vi "shippingM100.vi"() -> ()   [LabVIEW 2012]
uses:
  <vilib>/addons/database/Auxilliary.llb/DB Tools Cursor Type.ctl
  <vilib>/Utility/NIReport.llb/NI_report.lvclass
  <vilib>/addons/database/Connection.llb/DB Tools Open Connec (Path).vi
  <vilib>/addons/database/Connection.llb/Conn Execute.vi
  <vilib>/addons/database/Recordset.llb/Rec Destroy - Connection.vi
  <vilib>/addons/database/NI_Database_API.lvlib
panel:
  out "error out 2":errorcluster
  out "error out 4":errorcluster
  out "String 3":string
  out "String 2":string
  out "appended path":path
  out "size(s)":i32
  out "error out":errorcluster
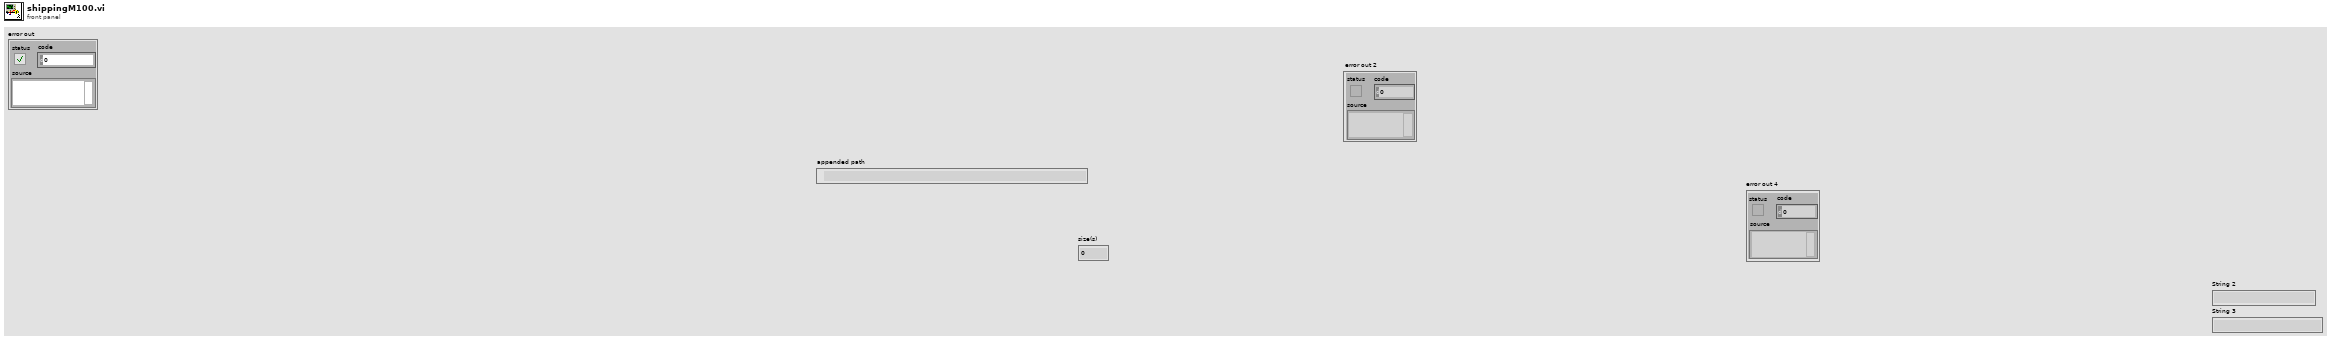
[diagram p1: front panel]
types:
  T1 = typedef "NI_Database_API.lvlib/DB Tools Cursor Type.ctl" = enum16{"forward-only", "keyset", "dynamic", "static"}
  T2 = typedef "NI_Database_API.lvlib/Conn ObjectReference.ctl" = refnum<k1>
  T3 = typedef "NI_Database_API.lvlib/Rec ObjectReference.ctl" = refnum<k1>
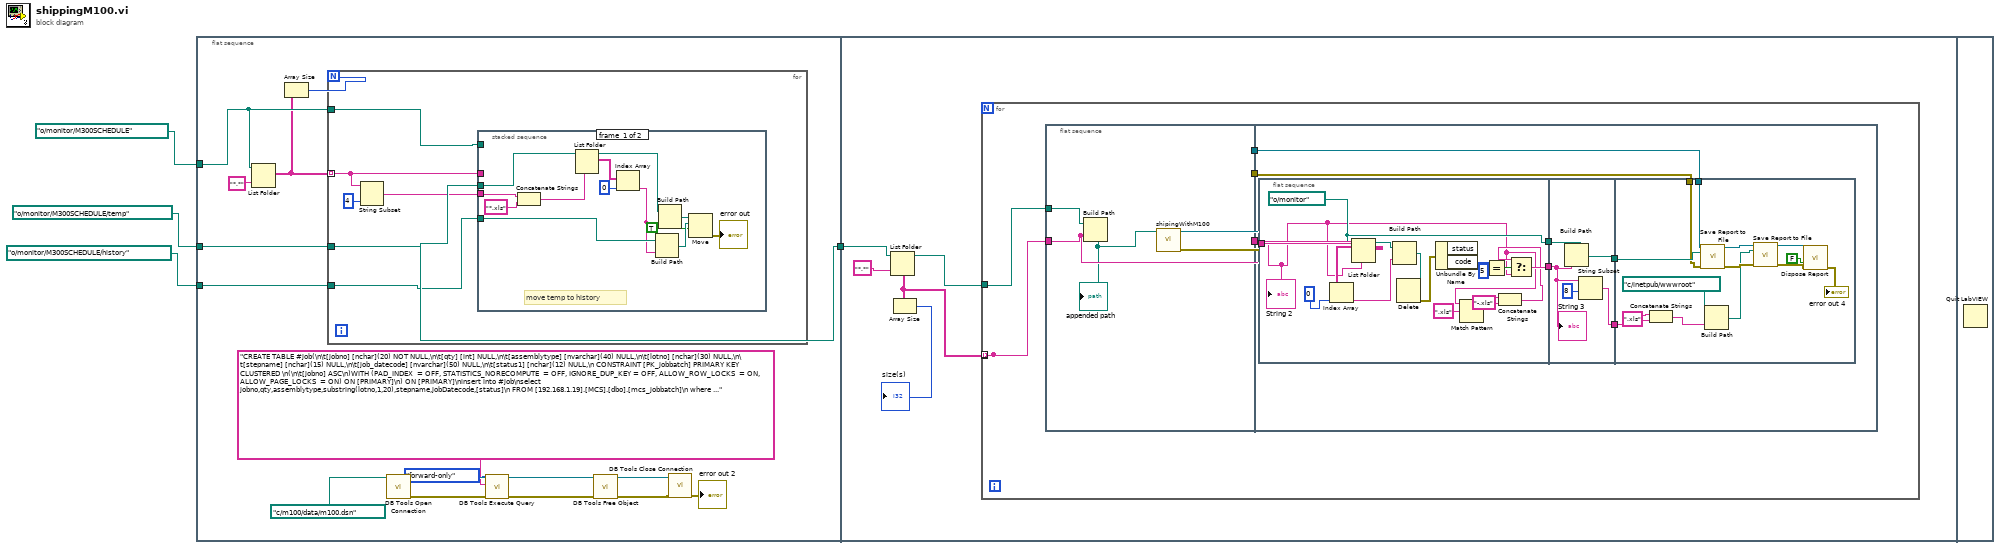
[diagram p0: block diagram]
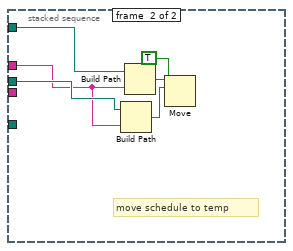
[diagram p2: hidden frame]
diagram:
  n1 = flat-sequence {
    tunnel: path "o:/monitor/M300SCHEDULE/temp" ("path") -> [w17]
    tunnel: [w17] -> w4
    tunnel: path "o:/monitor/M300SCHEDULE" ("path") -> [w19]
    tunnel: path "o:/monitor/M300SCHEDULE/history" ("path") -> [w18]
    tunnel: w4 -> [w49]
    frame #0 {
      n2 = List Folder(path=w19, pattern="*.*") -> (filenames=w15:string[])  [unwired: 2 in, 3 out]
      n3 = Array Size(array=w15) -> (size(s)=w16:i32)
      n4 = for {
        N: w16 -> [_]
        tunnel: w19 -> [w26]
        tunnel: w18 -> [w25]
        tunnel: w17 -> [w24]
        tunnel: w15 -> [w21] mode=indexing
        n5 = String Subset(string=w21, length (rest)=4 ("length (rest)")) -> (substring=w22:string)  [unwired: 1 in]
        n6 = stacked-sequence {
          tunnel: w24 -> [w35 w42]
          tunnel: w25 -> [w38 _]
          tunnel: w26 -> [_ w43]
          tunnel: w22 -> [w30 _]
          tunnel: w21 -> [_ w40]
          frame #0 {
            # "move temp to history"
            n7 = Concatenate Strings(w30, "*.xls" ("pattern")) -> (w28:string)
            n8 = List Folder(path=w35, pattern=w28) -> (path out=w34:path, filenames=w33:string[])  [unwired: 2 in, 2 out]
            n9 = Index Array(array=w33, index=0) -> (element=w31:string)
            n10 = Build Path(base path=w38, name or relative path=w31) -> (appended path=w37:path)
            n11 = Build Path(base path=w34, name or relative path=w31) -> (appended path=w39:path)
            n12 = Move(source path=w39, 9:TRUE ("overwrite (F)"), 10:w37) -> (error out=→"error out":errorcluster)  [unwired: 2 in, 2 out]
          }
          frame #1 {
            # "move schedule to temp"
            n13 = Build Path(base path=w42, name or relative path=w40) -> (appended path=w44:path)
            n14 = Build Path(base path=w43, name or relative path=w40) -> (appended path=w45:path)
            n15 = Move(source path=w45, 9:TRUE ("overwrite (F)"), 10:w44) -> ()  [unwired: 2 in, 3 out]
          }
        }
      }
      n16 = call-poly <vilib>:"DB Tools Open Connection.vi"("connection information"=path "c:/m100/data/m100.dsn") -> ("error out"=w12:errorcluster, "connection reference"=w14:T2)  [unwired: 7 in]
      n17 = call-poly <vilib>:"DB Tools Execute Query.vi"("error in (no error)"=w12, "cursor type"=DB_Tools_Cursor_Type."forward-only", "SQL query"="CREATE TABLE #job(\n\t[jobno] [nchar](20) NOT NULL,\n\t[qty] [int] NULL,\n\t[assemblytype] [nvarchar](40) NULL,\n\t[lotno] [nchar](30) NULL,\n\t[stepname] [nchar](15) NULL,\n\t[job_datecode] [nvarchar](50) NULL,\n\t[status1] [nchar](12) NULL,\n CONSTRAINT [PK_jobbatch] PRIMARY KEY CLUSTERED \n(\n\t[jobno] ASC\n)WITH (PAD_INDEX  = OFF, STATISTICS_NORECOMPUTE  = OFF, IGNORE_DUP_KEY = OFF, ALLOW_ROW_LOCKS  = ON, ALLOW_PAGE_LOCKS  = ON) ON [PRIMARY]\n) ON [PRIMARY]\ninsert into #job\nselect jobno,qty,assemblytype,substring(lotno,1,20),stepname,jobDatecode,[status]\n FROM [192.168.1.19].[MCS].[dbo].[mcs_jobbatch]\n where jobno not like '%M14110001%'\n   and lastupdatedate > 20140601", "connection reference"=w14) -> ("error out"=w11:errorcluster, "recordset reference"=w13:T3)  [unwired: 4 in]
      n18 = call-poly <vilib>:"DB Tools Free Object.vi"("error in (no error)"=w11, "recordset reference"=w13) -> ("error out"=w6:errorcluster, "connection reference"=w7:T2)  [unwired: 8 in]
      n19 = call <vilib>:"DB Tools Close Connection.vi"("error in (no error)"=w6, "connection reference"=w7) -> ("error out"=→"error out 2":errorcluster)  [unwired: 5 in]
    }
    frame #1 {
      n20 = List Folder(path=w49, pattern="*.*") -> (path out=w47:path, filenames=w46:string[])  [unwired: 2 in, 2 out]
      n21 = Array Size(array=w46) -> (size(s)=→"size(s)":i32)
      n22 = for {
        tunnel: w46 -> [w51] mode=indexing
        tunnel: [w51] -> _ mode=indexing
        tunnel: w47 -> [w55]
        n23 = flat-sequence {
          tunnel: w55 -> [w60]
          tunnel: w51 -> [w59]
          tunnel: [w59] -> w54
          tunnel: [w57] -> w53
          tunnel: [w56] -> w52
          tunnel: w54 -> [w64]
          tunnel: w53 -> [w63]
          tunnel: w52 -> [w62]
          frame #0 {
            n24 = Build Path(base path=w60, name or relative path=w59) -> (appended path=w58:path)
            "appended path" <- w58
            n25 = call "shipingWithM100.vi"("template (empty)"=w58) -> ("error out"=w56:errorcluster, "report out"=w57:refnum<class "NI_report.lvclass">)  [unwired: 9 in]
          }
          frame #1 {
            n26 = flat-sequence {
              tunnel: [w69] -> w67
              tunnel: [w71] -> w66
              tunnel: w64 -> [w68]
              tunnel: w67 -> [w88]
              tunnel: w66 -> [w87]
              tunnel: [w85] -> w65
              tunnel: [w84] -> w61
              tunnel: w65 -> [w100]
              tunnel: w63 -> [w99]
              tunnel: w62 -> [w98]
              tunnel: w61 -> [w91]
              frame #0 {
                w69 = path "o:/monitor" ("base path")
                n27 = List Folder(path=w69, pattern=w68) -> (path out=w81:path, filenames=w83:string[])  [unwired: 2 in, 2 out]
                n28 = Index Array(array=w83, index=0) -> (element=w80:string)
                n29 = Build Path(base path=w81, name or relative path=w80) -> (appended path=w79:path)
                n30 = Delete(path (use dialog)=w79) -> (error out=w78:errorcluster)  [unwired: 4 in, 2 out]
                n31 = Unbundle By Name(w78) -> ("code"=w77:i32)  [unwired: 1 out]
                n32 = Match Pattern(string=w68, regular expression=".xls") -> (match substring=w73:string)  [unwired: 1 in, 3 out]
                n33 = Equal?(x=w77, y=5) -> (x = y?=w75:bool)
                n34 = Concatenate Strings(w73, "-.xls" ("string")) -> (w70:string)
                n35 = Select(t=w70, s=w75, f=w68) -> (s? t:f=w71:string)
                "String 2" <- w68
              }
              frame #1 {
                n36 = Build Path(base path=w88, name or relative path=w87) -> (appended path=w85:path)
                n37 = String Subset(string=w87, length (rest)=8 ("length (rest)")) -> (substring=w84:string)  [unwired: 1 in]
                "String 3" <- w87
              }
              frame #2 {
                n38 = Concatenate Strings(w91, ".xls" ("string")) -> (w89:string)
                n39 = call-dynamic "Save Report to File.vi"("report in"=w99, "report file path"=w100, "error in (no error)"=w98) -> ("report out"=w95:refnum<class "NI_report.lvclass">, "error out"=w96:errorcluster)  [unwired: 11 in]
                n40 = Build Path(base path=path "c:/inetpub/wwwroot", name or relative path=w89) -> (appended path=w92:path)
                n41 = call-dynamic "Save Report to File.vi"("report in"=w95, "report file path"=w92, "error in (no error)"=w96) -> ("report out"=w94:refnum<class "NI_report.lvclass">, "error out"=w93:errorcluster)  [unwired: 11 in]
                n42 = call-dynamic "Dispose Report.vi"("report in"=w94, "save changes? (F)"=FALSE, "error in (no error)"=w93) -> ("error out"=→"error out 4":errorcluster)  [unwired: 12 in]
              }
            }
          }
        }
      }
    }
    frame #2 {
      n43 = Quit LabVIEW() -> ()  [unwired: 1 in]
    }
  }
